vi "Get Plot ID.vi"(8 "error in (no error)":errorcluster, 11 "3D Plot Datatype.lvclass in":refnum<class "3D Plot Datatype.lvclass">) -> (0 "error out":errorcluster, 1 "Plot ID":i32, 3 "3D Plot Datatype.lvclass out":refnum<class "3D Plot Datatype.lvclass">)   [LabVIEW 2017, in "3D Plot Datatype.lvclass"]
uses:
  <vilib>/Math Plots/3D Math Plots/3D Plot/3D Plot Datatype/3D Plot Datatype.lvclass
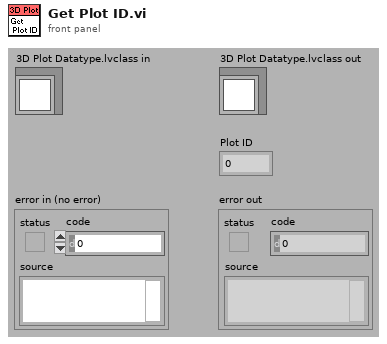
[diagram p1: front panel]
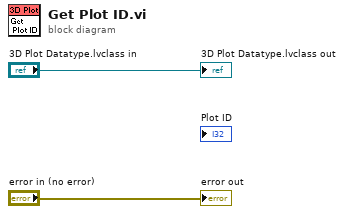
[diagram p0: block diagram]
diagram:
  "3D Plot Datatype.lvclass out" <- "3D Plot Datatype.lvclass in"
  "error out" <- "error in (no error)"
